vi "Start Experiment.vi"(8 "error in (no error)":errorcluster, 11 "ExperimentService in":refnum<class "ExperimentService.lvclass">) -> (0 "error out":errorcluster, 3 "ExperimentService out":refnum<class "ExperimentService.lvclass">)   [LabVIEW 2014, in "ExperimentService.lvclass"]
uses:
  ExperimentService.lvclass
  ExperimentService.lvclass/ExperimentService.ctl
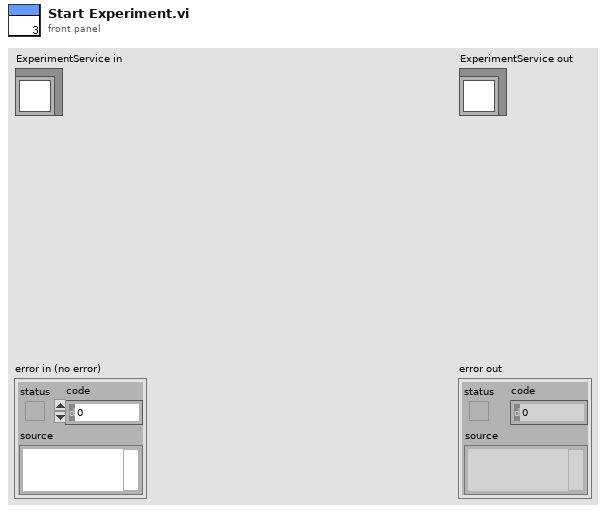
[diagram p1: front panel]
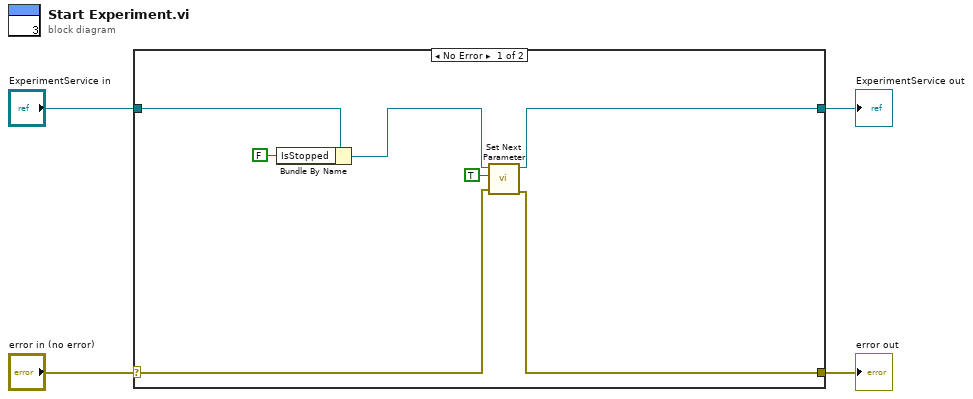
[diagram p0: block diagram]
diagram:
  n1 = case shown="No Error" "error in (no error)" {
    selector: "error in (no error)" -> [w9 w13]
    tunnel: [w10 w13] -> w3
    tunnel: [w11 w12] -> w1
    tunnel: "ExperimentService in" -> [w7 w12]
    frame No Error {
      n2 = Bundle By Name(cluster=w7, "IsStopped"=FALSE) -> (w6:refnum<class "ExperimentService.lvclass">)
      n3 = call-dynamic "Set Next Parameter.vi"("error in (no error)"=w9, "first?"=TRUE, "ExperimentService in"=w6) -> ("error out"=w10:errorcluster, "ExperimentService out"=w11:refnum<class "ExperimentService.lvclass">)  [unwired: 7 in]
    }
    frame Error {
    }
  }
  "error out" <- w3
  "ExperimentService out" <- w1
